vi "Filter Mappings.vi"(8 "error in (no error)":errorcluster, 9 "Path to Filter":string, 10 "Destinations":string[](array[string]), 11 "Sources":string[](array[string])) -> (0 "error out":errorcluster, 2 "Filtered Destinations":string[](array[string]), 3 "Filtered Sources":string[](array[string]))   [LabVIEW 2016, in "System Mapping Tool.lvlib"]
uses:
  System Mapping Tool.lvlib
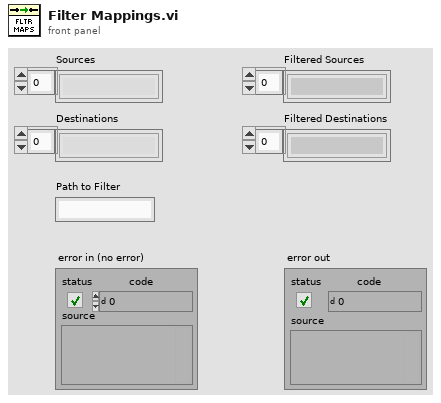
[diagram p1: front panel]
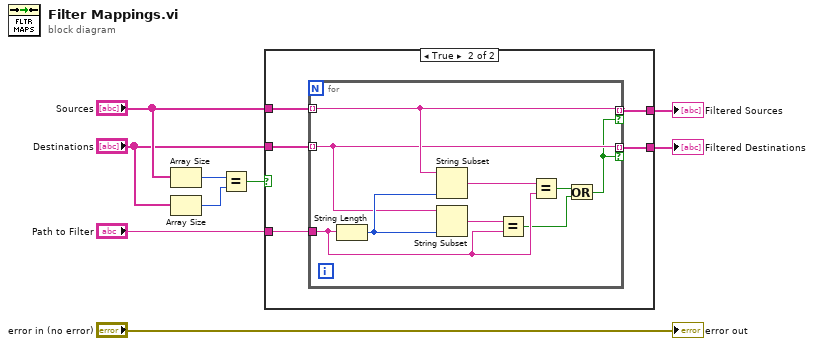
[diagram p0: block diagram]
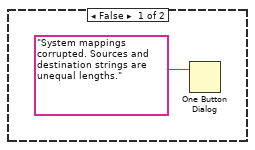
[diagram p2: hidden frame]
diagram:
  n1 = Array Size(array="Sources") -> (size(s)=w9:i32)
  n2 = Array Size(array="Destinations") -> (size(s)=w8:i32)
  n3 = Equal?(x=w9, y=w8) -> (x = y?=w7:bool)
  n4 = case shown="True" w7 {
    tunnel: "Sources" -> [_ w15]
    tunnel: "Destinations" -> [_ w14]
    tunnel: "Path to Filter" -> [_ w13]
    tunnel: [_ w12] -> w3
    tunnel: [_ w11] -> w2
    frame False {
      n5 = One Button Dialog(message="System mappings corrupted. Sources and destination strings are unequal lengths.") -> ()  [unwired: 1 in, 1 out]
    }
    frame True {
      n6 = for {
        tunnel: w15 -> [w18] mode=indexing
        tunnel: w14 -> [w17] mode=indexing
        tunnel: w13 -> [w21]
        tunnel: [w18] -> w11 mode=indexing if=w16
        tunnel: [w17] -> w12 mode=indexing if=w16
        n7 = String Length(string=w21) -> (length=w24:i32)
        n8 = String Subset(string=w18, length (rest)=w24) -> (substring=w22:string)  [unwired: 1 in]
        n9 = String Subset(string=w17, length (rest)=w24) -> (substring=w23:string)  [unwired: 1 in]
        n10 = Equal?(x=w23, y=w21) -> (x = y?=w19:bool)
        n11 = Equal?(x=w22, y=w21) -> (x = y?=w20:bool)
        n12 = Or(x=w20, y=w19) -> (x .or. y?=w16:bool)
      }
    }
  }
  "Filtered Sources" <- w2
  "Filtered Destinations" <- w3
  "error out" <- "error in (no error)"
